vi "Initiate_uC_connection.vi"(10 "reference in":refnum<vi>, 11 "VISAResourceName in":refnum<vi>) -> (3 "Array":string[](array[string]))   [LabVIEW 2020]
uses:
  <vilib>/Instr/_visa.llb/VISA Configure Serial Port (Instr).vi
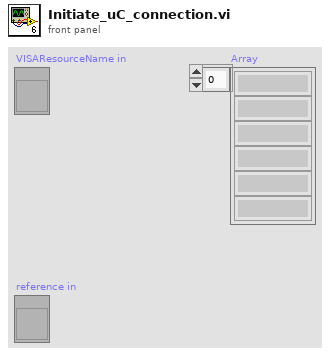
[diagram p1: front panel]
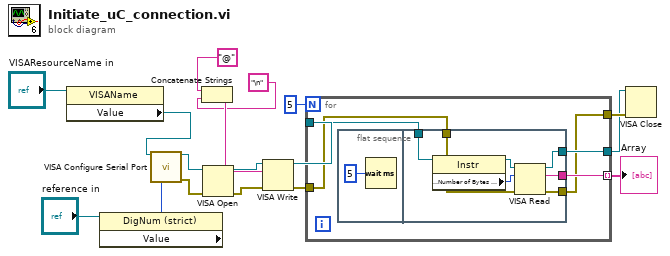
[diagram p0: block diagram]
diagram:
  n1 = property class="VISAName"(reference="VISAResourceName in") -> ("Value"=w4:refnum<visa-resource-name>)  [unwired: 1 in, 2 out]
  n2 = property class="DigNum (strict)"(reference="reference in") -> ("Value"=w3:u32)  [unwired: 1 in, 2 out]
  n3 = call-poly "VISA Configure Serial Port"("VISA resource name"=w4, "baud rate (9600)"=w3) -> ("VISA resource name out"=w6:refnum<visa-resource-name>, "error out"=w5:errorcluster)  [unwired: 12 in]
  n4 = Concatenate Strings("@" ("String"), "\n") -> (w11:string)
  n5 = VISA Open(error in (no error)=w5, VISA resource name=w6) -> (VISA resource name=w8:refnum<visa-resource-name>, error out=w12:errorcluster)  [unwired: 3 in]
  n6 = VISA Write(VISA resource name=w8, write buffer=w11, error in (no error)=w12) -> (VISA resource name out=w13:refnum<visa-resource-name>, error out=w7:errorcluster)  [unwired: 1 out]
  n7 = for {
    N: 5 -> [_]
    tunnel: w7 -> [w21]
    tunnel: w13 -> [w22]
    tunnel: [w20] -> w14 mode=indexing
    tunnel: [w19] -> w15
    tunnel: [w18] -> w16
    n8 = flat-sequence {
      tunnel: w22 -> [w29]
      tunnel: w21 -> [w30]
      tunnel: [w27] -> w20
      tunnel: [w26] -> w19
      tunnel: [w25] -> w18
      frame #0 {
        n9 = Wait (ms)(milliseconds to wait=u32 5) -> ()  [unwired: 1 out]
      }
      frame #1 {
        n10 = property class="Instr"(reference=w29) -> (reference out=w28:refnum<visa-resource-name>, "Serial Settings:Number of Bytes at Serial Port"=w24:u32)  [unwired: 1 in, 1 out]
        n11 = VISA Read(VISA resource name=w28, byte count=w24, error in (no error)=w30) -> (VISA resource name out=w26:refnum<visa-resource-name>, read buffer=w27:string, error out=w25:errorcluster)  [unwired: 1 out]
      }
    }
  }
  "Array" <- w14
  n12 = VISA Close(VISA resource name=w15, error in (no error)=w16) -> ()  [unwired: 1 out]
